vi "UpdatePos.vi"(10 "Direction":T1, 11 "Atom In":refnum<class "Atom.lvclass">) -> (3 "Atom Out":refnum<class "Atom.lvclass">)   [LabVIEW 2017, in "Atom.lvclass"]
uses:
  Atom.lvclass
  Type Defs/Direction Enum.ctl
  Atom.lvclass/Atom.ctl
  Type Defs/SB Type Defs.lvlib
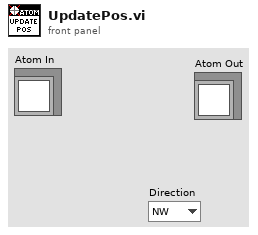
[diagram p1: front panel]
types:
  T1 = typedef "SB Type Defs.lvlib/Direction Enum.ctl" = enum16{"NW", "N", "NE", "E", "SE", "S", "SW", "W"}
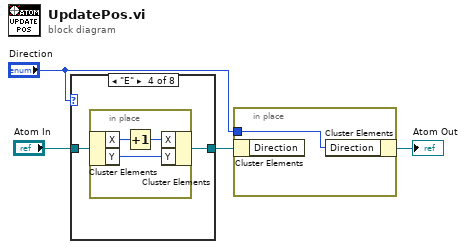
[diagram p0: block diagram]
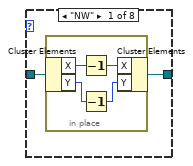
[diagram p2: hidden frame]
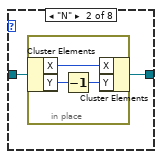
[diagram p3: hidden frame]
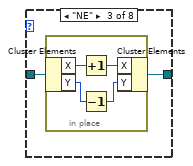
[diagram p4: hidden frame]
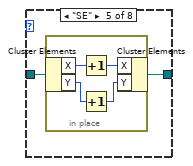
[diagram p5: hidden frame]
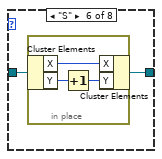
[diagram p6: hidden frame]
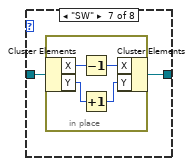
[diagram p7: hidden frame]
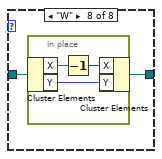
[diagram p8: hidden frame]
diagram:
  n1 = case shown="\"E\"" "Direction" {
    tunnel: [w6 w12 w17 w23 w28 w34 w39 w45] -> w3
    tunnel: "Atom In" -> [w5 w11 w16 w22 w27 w33 w38 w44]
    frame "NW" {
      n2 = in-place {
        n3 = in-place-cluster #1(w5) -> ("X"=w10:i32, "Y"=w8:i32)
        n4 = Decrement(x=w10) -> (x-1=w9:i32)
        n5 = Decrement(x=w8) -> (x-1=w7:i32)
        n6 = in-place-cluster #1("X"=w9, "Y"=w7) -> (w6:refnum<class "Atom.lvclass">)
      }
    }
    frame "N" {
      n7 = in-place {
        n8 = in-place-cluster #2(w11) -> ("X"=w15:i32, "Y"=w14:i32)
        n9 = Decrement(x=w14) -> (x-1=w13:i32)
        n10 = in-place-cluster #2("X"=w15, "Y"=w13) -> (w12:refnum<class "Atom.lvclass">)
      }
    }
    frame "NE" {
      n11 = in-place {
        n12 = in-place-cluster #3(w16) -> ("X"=w21:i32, "Y"=w20:i32)
        n13 = Increment(x=w21) -> (x+1=w18:i32)
        n14 = Decrement(x=w20) -> (x-1=w19:i32)
        n15 = in-place-cluster #3("X"=w18, "Y"=w19) -> (w17:refnum<class "Atom.lvclass">)
      }
    }
    frame "E" {
      n16 = in-place {
        n17 = in-place-cluster #4(w22) -> ("X"=w26:i32, "Y"=w25:i32)
        n18 = Increment(x=w26) -> (x+1=w24:i32)
        n19 = in-place-cluster #4("X"=w24, "Y"=w25) -> (w23:refnum<class "Atom.lvclass">)
      }
    }
    frame "SE" {
      n20 = in-place {
        n21 = in-place-cluster #5(w27) -> ("X"=w32:i32, "Y"=w31:i32)
        n22 = Increment(x=w32) -> (x+1=w30:i32)
        n23 = Increment(x=w31) -> (x+1=w29:i32)
        n24 = in-place-cluster #5("X"=w30, "Y"=w29) -> (w28:refnum<class "Atom.lvclass">)
      }
    }
    frame "S" {
      n25 = in-place {
        n26 = in-place-cluster #6(w33) -> ("X"=w37:i32, "Y"=w36:i32)
        n27 = Increment(x=w36) -> (x+1=w35:i32)
        n28 = in-place-cluster #6("X"=w37, "Y"=w35) -> (w34:refnum<class "Atom.lvclass">)
      }
    }
    frame "SW" {
      n29 = in-place {
        n30 = in-place-cluster #7(w38) -> ("X"=w43:i32, "Y"=w42:i32)
        n31 = Decrement(x=w43) -> (x-1=w40:i32)
        n32 = Increment(x=w42) -> (x+1=w41:i32)
        n33 = in-place-cluster #7("X"=w40, "Y"=w41) -> (w39:refnum<class "Atom.lvclass">)
      }
    }
    frame "W" {
      n34 = in-place {
        n35 = in-place-cluster #8(w44) -> ("X"=w48:i32, "Y"=w47:i32)
        n36 = Decrement(x=w48) -> (x-1=w46:i32)
        n37 = in-place-cluster #8("X"=w46, "Y"=w47) -> (w45:refnum<class "Atom.lvclass">)
      }
    }
  }
  n38 = in-place {
    in-place-border: "Direction" -> [w49]
    n39 = in-place-cluster #9(w3) -> ()  [unwired: 1 out]
    n40 = in-place-cluster #9("Direction"=w49) -> (→"Atom Out":refnum<class "Atom.lvclass">)
  }
